vi "Read Gate CO.vi"(8 "error in (no error)":errorcluster, 11 "cCRDS_new in":refnum<class "cCRDS.lvclass">=refnum) -> (0 "error out":errorcluster, 2 "Gate CO":refnum<k21>, 3 "cCRDS_new out":refnum<class "cCRDS.lvclass">)   [LabVIEW 2015, in "cCRDS.lvclass"]
uses:
  cCRDS.lvclass
  cCRDS.lvclass/cCRDS.ctl
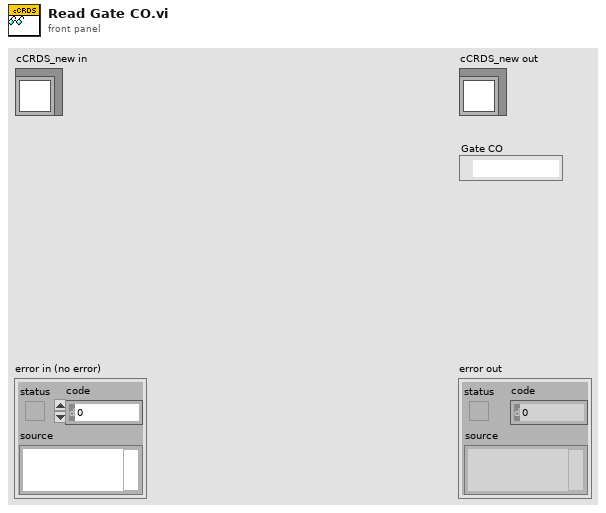
[diagram p1: front panel]
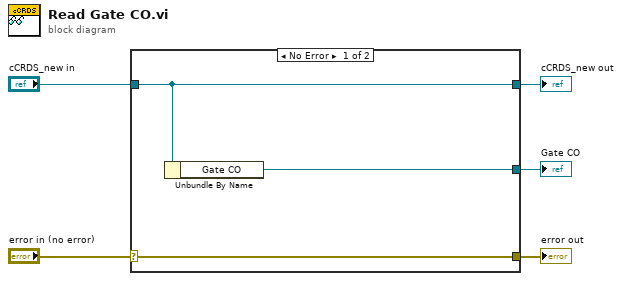
[diagram p0: block diagram]
diagram:
  n1 = case shown="No Error" "error in (no error)" {
    selector: "error in (no error)" -> [w8 w9]
    tunnel: [w8 w9] -> w4
    tunnel: [w7 w10] -> w2
    tunnel: "cCRDS_new in" -> [w7 w10]
    tunnel: [w6 _] -> w1
    frame No Error {
      n2 = Unbundle By Name(w7) -> ("Gate CO"=w6:refnum<k21>)
    }
    frame Error {
    }
  }
  "error out" <- w4
  "cCRDS_new out" <- w2
  "Gate CO" <- w1
